vi "Builder.Main.vi"(8 "error in (no error)":errorcluster, 11 "Builder in":refnum<class "Builder.lvclass">) -> (0 "error out":errorcluster, 3 "Builder out":refnum<class "Builder.lvclass">)   [LabVIEW 2016, in "DSF.Engine.lvlib" / "Builder.lvclass"]
uses:
  Builder.lvclass
  Builder.lvclass/Builder.ctl
  Thread Parameters/Thread Parameters.lvclass/Thread Parameters.ctl
  <vilib>/Platform/TimedLoop/XDataNode/timing_clust.ctl
  <vilib>/Platform/TimedLoop/XDataNode/nitl_modes.ctl
  <vilib>/Platform/TimedLoop/XDataNode/wakeup.ctl
  Interface/DSF.Engine.Interface.lvclass/DSF.Engine.Interface.ctl
  Interface/DSF.Engine.Interface.Builder.Response Data.ctl
  Interface/DSF.Engine.Interface.Builder.Response.ctl
  Interface/DSF.Engine.Interface.Builder.Read.Command.vi
  Interface/DSF.Engine.Interface.Builder.Write.Response.vi
  Interface/DSF.Engine.Interface.Get Command FIFO.vi
  Interface/DSF.Engine.Interface.RT FIFO.Read.vi
  Interface/DSF.Engine.Interface.RT FIFO.Write.vi
  Interface/DSF.Engine.Interface.Builder.lvclass
  C:/Git/Sourcetree/DSF/Source/Engine/Classes/Interface/DSF.Engine.Interface.lvclass
  <vilib>/platform/TimedLoop/XDataNode/XDataNode.xnode
  Thread Parameters/Thread Parameters.lvclass
  <vilib>/Platform/TimedLoop/XDataNode/XDNodeRunTimeDep.lvlib
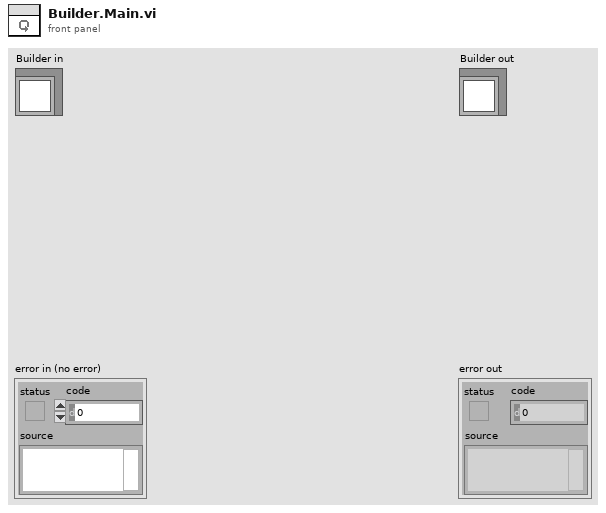
[diagram p1: front panel]
types:
  T1 = typedef "XDNodeRunTimeDep.lvlib/timing_clust.ctl" = cluster{"Expected End [f-1]":u64, "Actual End [f-1]":u64, "Finished Late? [f-1]":bool, "Expected End [i-1]":u64, "Actual End [i-1]":u64, "Finished Late? [i-1]":bool, "Expected Start [i]":u64, "Actual Start [i]":u64, "Expected Start [f]":u64, "Actual Start [f]":u64, "Source Name":string, "Structure Name":string, "Period":i64, "Deadline":i64, "Offset":i64, "Start":i64, "Priority":i32, "Timeout":i32, "Mode":T2, "Wakeup Reason":T3, "Error":errorcluster, "Source Type":string, "Secondary Source Type":string, "Global End Time":u64, "Global Start Time":u64, "Frame Duration":u64, "Iteration Duration":u64, "Assigned CPU":i32, "I/O Scan Engine Mode":u32}
  T2 = typedef "XDNodeRunTimeDep.lvlib/nitl_modes.ctl" = enum32{"No Change", "Process missed periods, maintain original phase", "Discard missed periods, maintain original phase", "Process missed periods, ignore original phase", "Discard missed periods, ignore original phase"}
  T3 = typedef "XDNodeRunTimeDep.lvlib/wakeup.ctl" = enum32{"Normal", "Aborted", "Asynchronous wakeup", "Timing source error", "Timed loop error", "Timeout"}
  T4 = typedef "DSF.Engine.lvlib/DSF.Engine.Interface.Builder.lvclass/DSF.Engine.Interface.Builder.Response Data.ctl" = cluster{"Response":T5, "Payload":u64}
  T5 = typedef "DSF.Engine.lvlib/DSF.Engine.Interface.Builder.lvclass/DSF.Engine.Interface.Builder.Response.ctl" = enum8{"General Ack", "Shutdown Ack"}
  T6 = typedef "DSF.Engine.lvlib/DSF.Engine.Interface.Builder.lvclass/DSF.Engine.Interface.Builder.Command Data.ctl" = cluster{"Command":T7, "Payload":u64}
  T7 = typedef "DSF.Engine.lvlib/DSF.Engine.Interface.Builder.lvclass/DSF.Engine.Interface.Builder.Command.ctl" = enum8{"Idle", "Initialize", "Build Buffer", "Parse Buffer", "Shutdown"}
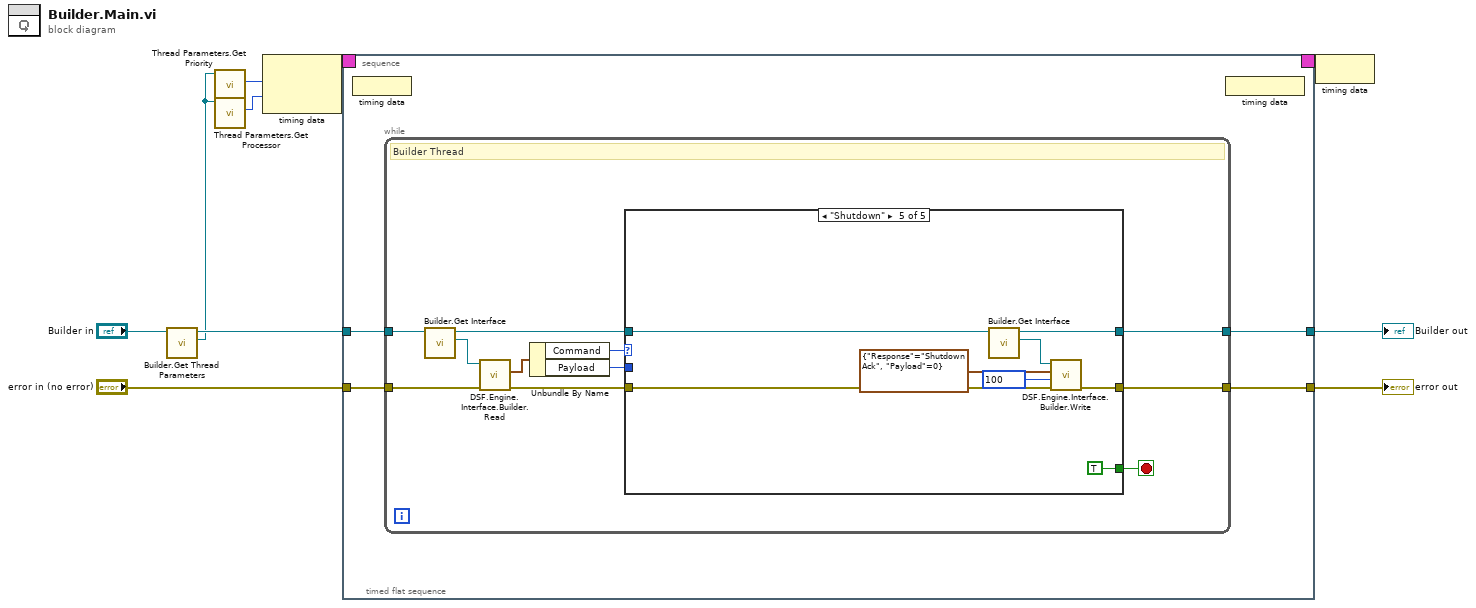
[diagram p0: block diagram]
diagram:
  n1 = call "Builder.Get Thread Parameters.vi"("Builder in"="Builder in") -> ("Thread Parameters"=w2:refnum<class "Thread Parameters.lvclass">, "Builder out"=w7:refnum<class "Builder.lvclass">)  [unwired: 9 in]
  n2 = call "Thread Parameters.Get Priority.vi"("Thread Parameters in"=w2) -> ("Priority"=w6:i32)  [unwired: 9 in, 1 out]
  n3 = call "Thread Parameters.Get Processor.vi"("Thread Parameters in"=w2) -> ("Processor"=w5:i32)  [unwired: 9 in, 1 out]
  n4 = node-c288(w6, w5) -> (w9:T1)
  n5 = timed-sequence {
    timing: w9 -> [_]
    timing-out: [_] -> w8
    tunnel: w7 -> [w13]
    tunnel: [w14] -> w4
    tunnel: "error in (no error)" -> [w12]
    tunnel: [w11] -> w1
    n6 = timed-flat-sequence {
      tunnel: [w18] -> w14
      tunnel: w13 -> [w16]
      tunnel: w12 -> [w17]
      tunnel: [w15] -> w11
      n7 = node-c288() -> ()  [unwired: 1 in]
      n8 = while {
        tunnel: w16 -> [w22]
        tunnel: [w26] -> w18
        tunnel: w17 -> [w30]
        tunnel: [w23] -> w15
        stop <- w21 stop-if-true
        # "Builder Thread"
        n9 = call "Builder.Get Interface.vi"("Builder in"=w22) -> ("Builder Interface"=w31:refnum<class "DSF.Engine.Interface.Builder.lvclass">, "Builder out"=w27:refnum<class "Builder.lvclass">)  [unwired: 9 in]
        n10 = call-poly "DSF.Engine.Interface.Builder.Read.vi"("error in (no error)"=w30, "Builder Interface in"=w31) -> ("error out"=w24:errorcluster, "command"=w29:T6)  [unwired: 5 in, 3 out]
        n11 = Unbundle By Name(w29) -> ("Command"=w28:T7, "Payload"=w25:u64)
        n12 = case shown="\"Shutdown\"" w28 {
          tunnel: w27 -> [w33 w35 w37 w39 w47]
          tunnel: [w33 w35 w37 w39 w46] -> w26
          tunnel: w25 -> [_ _ _ _ _]
          tunnel: w24 -> [w32 w34 w36 w38 w42]
          tunnel: [w32 w34 w36 w38 w45] -> w23
          tunnel: [_ _ _ _ TRUE] -> w21
          frame "Idle", Default {
          }
          frame "Initialize" {
          }
          frame "Build Buffer" {
          }
          frame "Parse Buffer" {
          }
          frame "Shutdown" {
            n13 = call "Builder.Get Interface.vi"("Builder in"=w47) -> ("Builder Interface"=w44:refnum<class "DSF.Engine.Interface.Builder.lvclass">, "Builder out"=w46:refnum<class "Builder.lvclass">)  [unwired: 9 in]
            n14 = call-poly "DSF.Engine.Interface.Builder.Write.vi"("error in (no error)"=w42, "timeout in ms (0)"=100, "response"=T4 {"Response"=enum."Shutdown Ack", "Payload"=0}, "Builder Interface in"=w44) -> ("error out"=w45:errorcluster)  [unwired: 5 in, 2 out]
          }
        }
      }
      n15 = node-c288() -> ()  [unwired: 1 out]
    }
  }
  "error out" <- w1
  "Builder out" <- w4
  n16 = node-c288(w8) -> ()
